vi "RSZVB Get Low Phase Noise State.vi"(8 "error in (no error)":errorcluster {"code" format="%.0x"}, 10 "Channel (1)":i32=1, 11 "VISA session":refnum<visa-resource-name>) -> (0 "error out":errorcluster {"code" format="%.0x"}, 2 "Low Phase Noise State":bool, 3 "dup VISA session":refnum<visa-resource-name>)   [LabVIEW 2011]
doc: "This VI returns the state of the Low Phase Noise VI. \n\nRemote-control command(s):\n[SENSe<Ch>:]FREQuency:LPNoise <Boolean>"
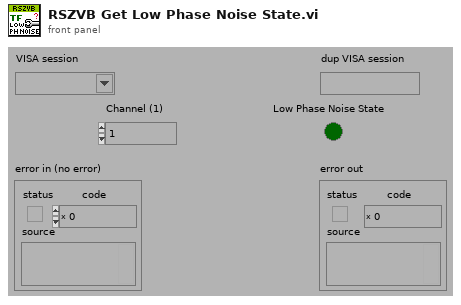
[diagram p1: front panel]
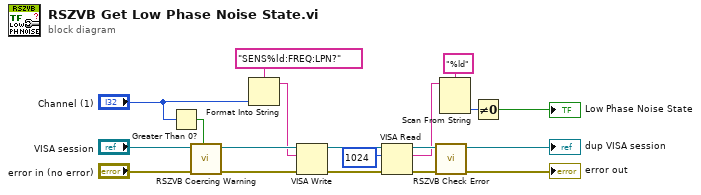
[diagram p0: block diagram]
diagram:
  n1 = Greater Than 0?(x="Channel (1)") -> (x > 0?=w15:bool)
  n2 = call "RSZVB Coercing Warning.vi"("In Range?"=w15, "error in (no error)"="error in (no error)", "VISA session"="VISA session") -> ("error out"=w17:errorcluster, "dup VISA session"=w18:refnum<visa-resource-name>)  [unwired: 7 in]
  n3 = Format Into String(format string="SENS%ld:FREQ:LPN?", "Channel (1)") -> (resulting string=w16:string)  [unwired: 2 in, 1 out]
  n4 = VISA Write(VISA resource name=w18, write buffer=w16, error in (no error)=w17) -> (VISA resource name out=w10:refnum<visa-resource-name>, error out=w11:errorcluster)  [unwired: 1 out]
  n5 = VISA Read(VISA resource name=w10, byte count=u32 1024 ("byte count (0)"), error in (no error)=w11) -> (VISA resource name out=w13:refnum<visa-resource-name>, read buffer=w9:string, error out=w12:errorcluster)  [unwired: 1 out]
  n6 = call "RSZVB Check Error.vi"("error in (no error)"=w12, "VISA session"=w13) -> ("error out"=→"error out":errorcluster, "dup VISA session"=→"dup VISA session":refnum<visa-resource-name>)  [unwired: 8 in]
  n7 = Scan From String(format string="%ld", input string=w9) -> (output 1=w7:i32)  [unwired: 3 in, 3 out]
  n8 = Not Equal To 0?(x=w7) -> (x != 0?=→"Low Phase Noise State":bool)
